vi "Read Keys.vi"(7 "Prefix/Regex":enum16{"Prefix", "Regex"}(ring), 8 "error in (no error)":errorcluster, 10 "Selector":string, 11 "FlexWorktable in":refnum<class "FlexWorktable.lvclass">) -> (0 "error out":errorcluster, 2 "Keys":string[](array[string]), 3 "FlexWorktable out":refnum<class "FlexWorktable.lvclass">)   [LabVIEW 2017, in "FlexWorktable.lvclass"]
uses:
  FlexWorktable.lvclass
  FlexWorktable.lvclass/FlexWorktable.ctl
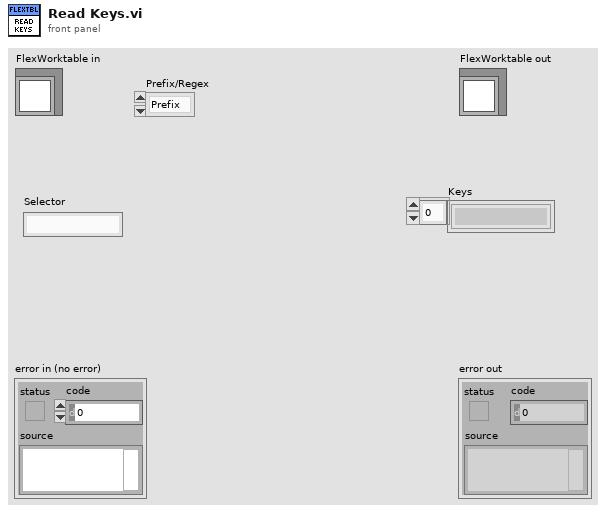
[diagram p1: front panel]
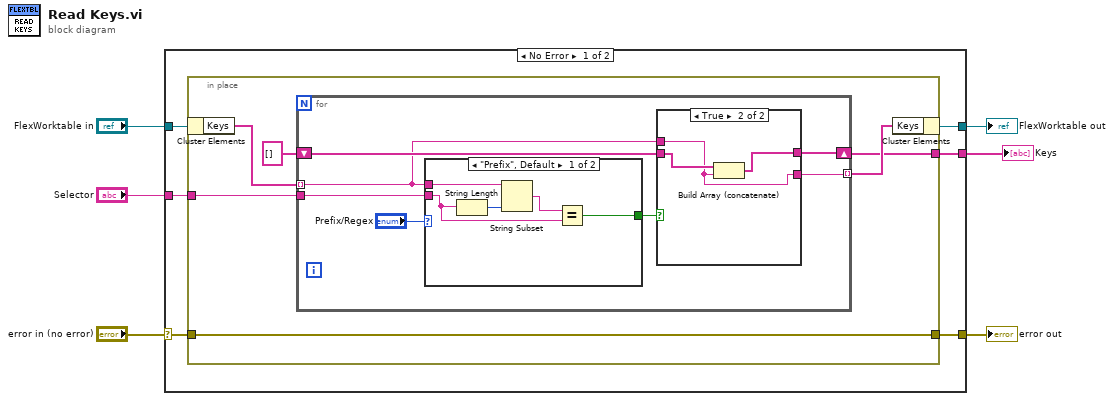
[diagram p0: block diagram]
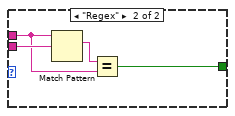
[diagram p2: hidden frame]
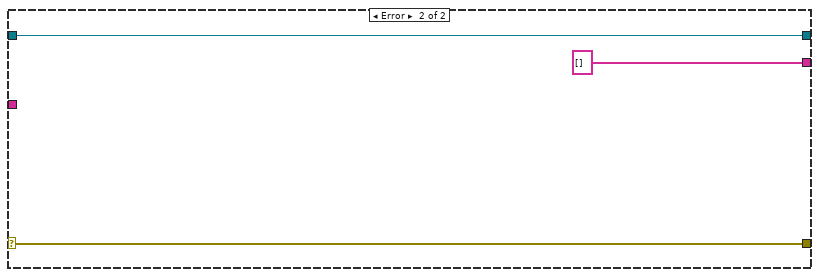
[diagram p4: hidden frame]
diagram:
  n1 = case shown="No Error" "error in (no error)" {
    selector: "error in (no error)" -> [w10 w42]
    tunnel: [w7 w42] -> w5
    tunnel: [w8 w41] -> w3
    tunnel: "FlexWorktable in" -> [w12 w41]
    tunnel: "Selector" -> [w11 _]
    tunnel: [w9 string[] [] ("Keys")] -> w1
    frame No Error {
      n2 = in-place {
        in-place-border: w11 -> [w16]
        in-place-border: w10 -> [w13]
        in-place-border: [w14] -> w9
        in-place-border: [w13] -> w7
        n3 = in-place-cluster #1(w12) -> ("Keys"=w18:string[])
        n4 = for {
          tunnel: w18 -> [w22] mode=indexing
          shift-right: [w21] -> w14
          shift-left: string[] [] ("Keys") -> [w23]
          tunnel: w16 -> [w25]
          tunnel: [w20] -> w15 mode=indexing
          n5 = case shown="\"Prefix\", Default" "Prefix/Regex" {
            tunnel: w25 -> [w27 w34]
            tunnel: [w26 w32] -> w24
            tunnel: w22 -> [w30 w31]
            frame "Prefix", Default {
              n6 = String Length(string=w27) -> (length=w29:i32)
              n7 = String Subset(string=w30, length (rest)=w29) -> (substring=w28:string)  [unwired: 1 in]
              n8 = Equal?(x=w28, y=w27) -> (x = y?=w26:bool)
            }
            frame "Regex" {
              n9 = Match Pattern(string=w31, regular expression=w34) -> (match substring=w33:string)  [unwired: 1 in, 3 out]
              n10 = Equal?(x=w33, y=w31) -> (x = y?=w32:bool)
            }
          }
          n11 = case shown="True" w24 {
            tunnel: w23 -> [w36 w39]
            tunnel: w22 -> [w35 w37]
            tunnel: [w36 w38] -> w21
            tunnel: [w35 w37] -> w20
            frame False {
            }
            frame True {
              n12 = Build Array (concatenate)(w39, w37) -> (w38:string[])
            }
          }
        }
        n13 = in-place-cluster #1("Keys"=w15) -> (w8:refnum<class "FlexWorktable.lvclass">)
      }
    }
    frame Error {
    }
  }
  "error out" <- w5
  "FlexWorktable out" <- w3
  "Keys" <- w1
